vi "Get Temperature Status.vi"(7 "CoolerVolts":sgl, 8 "error in (no error)":errorcluster, 9 "AmbientTemp":sgl, 10 "TargetTemp":sgl, 11 "SensorTemp":sgl) -> (0 "error out":errorcluster, 1 "AmbientTemp out":sgl, 2 "TargetTemp out":sgl, 3 "SensorTemp out":sgl, 4 "function return":u32, 5 "CoolerVolts out":sgl)   [LabVIEW 2018, in "AndorSDK.lvlib"]
doc: "EXPNETTYPE unsigned int WINAPI GetTemperatureStatus(float * SensorTemp, float * TargetTemp, float * AmbientTemp, float * CoolerVolts);"
uses:
  AndorSDK.lvlib
  ATMCD32D.dll
  OwnVIs/AndorOWN.lvlib
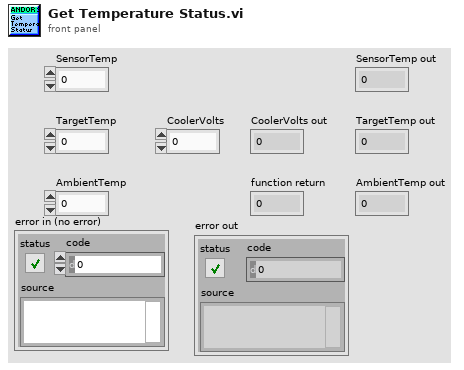
[diagram p1: front panel]
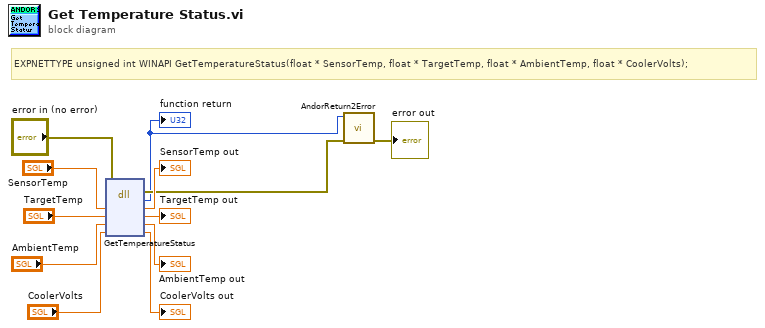
[diagram p0: block diagram]
diagram:
  # "EXPNETTYPE unsigned int WINAPI GetTemperatureStatus(float * SensorTemp, float * TargetTemp, float * AmbientTemp, float * CoolerVolts);"
  n1 = dll-call lib="C:/Users/e14user/Documents/LabVIEW software/GitRepo/lib/ANDOR/Andor SDK/ATMCD32D.*" fn="GetTemperatureStatus"(error in="error in (no error)", "SensorTemp"="SensorTemp", "TargetTemp"="TargetTemp", "AmbientTemp"="AmbientTemp", "CoolerVolts"="CoolerVolts") -> (error out=w3:errorcluster, w2:u32, "SensorTemp"=→"SensorTemp out":sgl, "TargetTemp"=→"TargetTemp out":sgl, "AmbientTemp"=→"AmbientTemp out":sgl, "CoolerVolts"=→"CoolerVolts out":sgl)  [unwired: 2 in, 1 out]
  "function return" <- w2
  n2 = call "AndorReturn2Error.vi"("error in (no error)"=w3, "Camera return"=w2) -> ("error out"=→"error out":errorcluster)  [unwired: 9 in]
